vi "ADC.vi"(0 "source":tag, 1 "physical channels":tag, 2 "rate":dbl=1000.0 format="%0.2f", 3 "error in":errorcluster, 4 "samples per channel":i32=1000) -> (5 "Waveform Graph":dbl[](graph), 6 "Fourier spectrum":dbl[](graph), 7 "error out":errorcluster)   [LabVIEW 2018]
uses:
  <vilib>/DAQmx/read.llb/DAQmx Read (Analog 1D DBL 1Chan NSamp).vi
  <vilib>/DAQmx/create/channels.llb/DAQmx Create Channel (AI-Voltage-Basic).vi
  <vilib>/DAQmx/configure/timing.llb/DAQmx Timing (Sample Clock).vi
  <vilib>/DAQmx/miscellaneous.llb/DAQmx Fill In Error Info.vi
  <vilib>/Analysis/NI_AALPro.lvlib
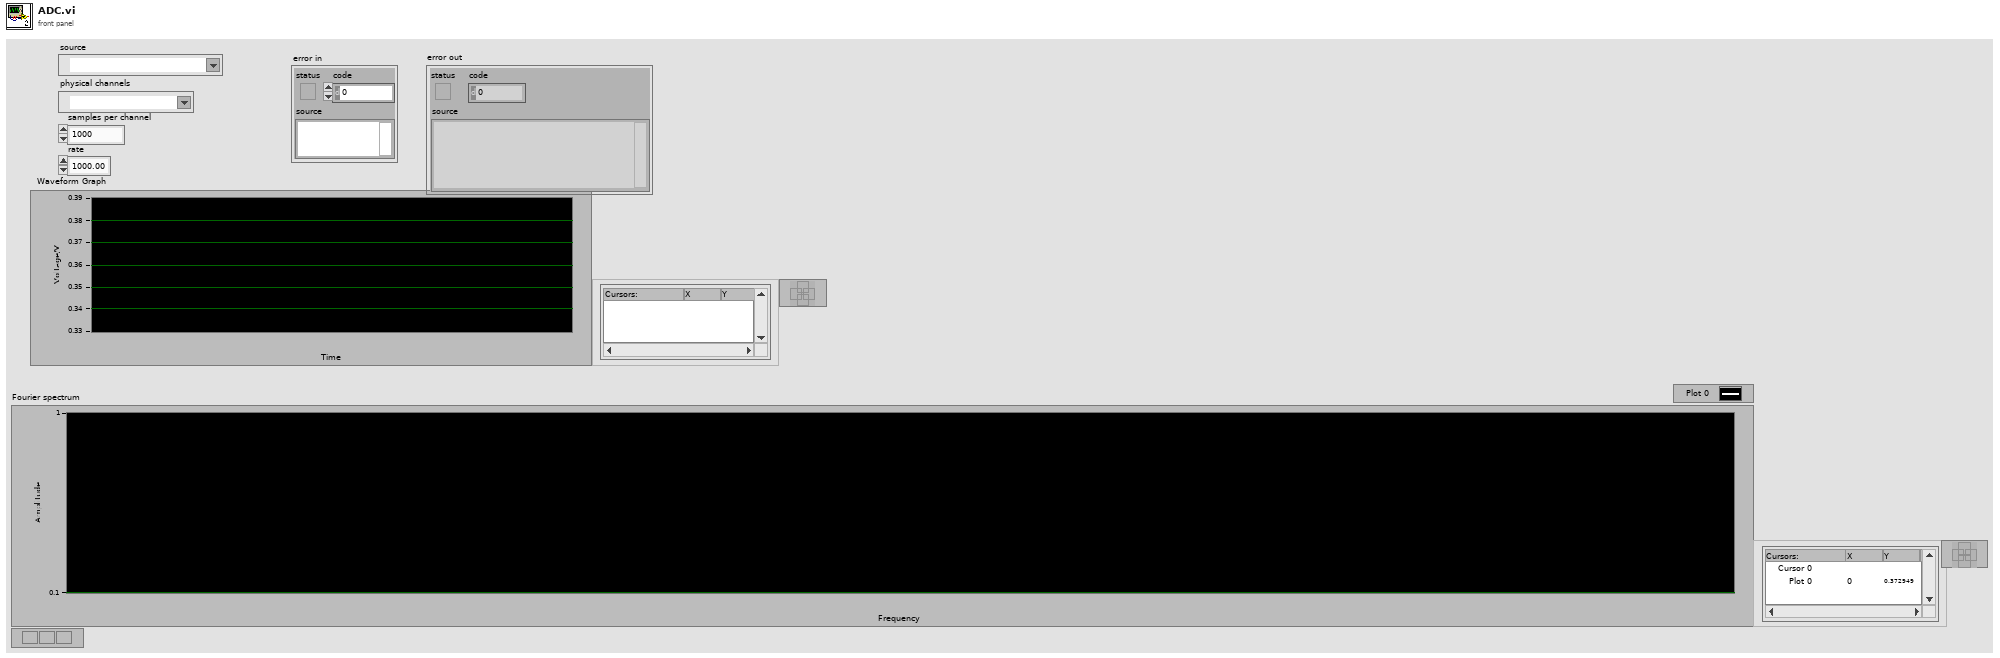
[diagram p1: front panel]
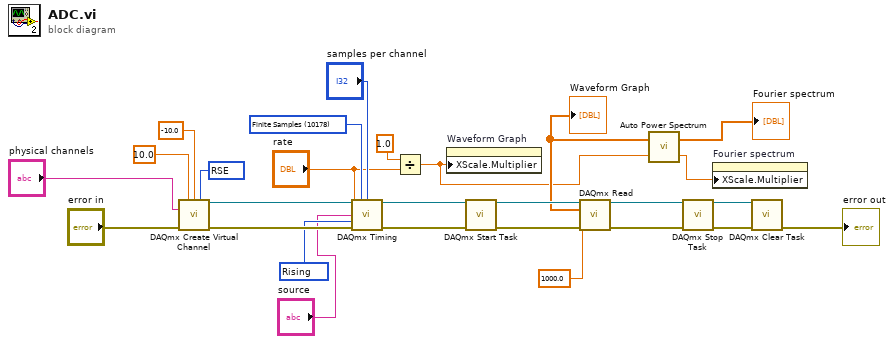
[diagram p0: block diagram]
diagram:
  w13 = 10083 items=["Default"=-1, "RSE"=10083, "NRSE"=10078, "Differential"=10106, "Pseudodifferential"=12529] ("input terminal configuration")
  w12 = 10280 items=["Rising"=10280, "Falling"=10171] ("active edge")
  w24 = 10178 items=["Finite Samples"=10178, "Continuous Samples"=10123, "Hardware Timed Single Point"=12522] ("sample mode")
  n1 = call-poly <vilib>:"DAQmx Create Virtual Channel.vi"("maximum value"=10.0, "minimum value"=-10.0, "input terminal configuration"=w13, "physical channels"="physical channels", "error in"="error in") -> ("task out"=w26:refnum<k21>, "error out"=w25:errorcluster)  [unwired: 9 in]
  n2 = call-poly <vilib>:"DAQmx Timing.vi"("task/channels in"=w26, "sample mode"=w24, "samples per channel"="samples per channel", "rate"="rate", "source"="source", "active edge"=w12, "error in"=w25) -> ("task out"=w23:refnum<k21>, "error out"=w22:errorcluster)  [unwired: 7 in]
  n3 = Divide(x=1.0, y="rate") -> (x/y=w7:dbl)
  n4 = property on="Waveform Graph" class="WFGraph (strict)"("XScale.Multiplier"=w7) -> ()  [unwired: 2 in, 2 out]
  n5 = call <vilib>:"DAQmx Start Task.vi"("task/channels in"=w23, "error in"=w22) -> ("task out"=w17:refnum<k21>, "error out"=w3:errorcluster)  [unwired: 12 in]
  n6 = call-poly <vilib>:"DAQmx Read.vi"("task/channels in"=w17, "timeout"=1000.0, "error in"=w3) -> ("task out"=w16:refnum<k21>, "data"=w8:dbl[], "error out"=w4:errorcluster)  [unwired: 10 in]
  "Waveform Graph" <- w8
  n7 = call <vilib>:"Auto Power Spectrum.vi"("dt"=w7, "Signal (V)"=w8) -> ("df"=w5:dbl, "Power Spectrum (V^2 rms)"=→"Fourier spectrum":dbl[])
  n8 = call <vilib>:"DAQmx Stop Task.vi"("task/channels in"=w16, "error in"=w4) -> ("task out"=w21:refnum<k21>, "error out"=w20:errorcluster)  [unwired: 12 in]
  n9 = property on="Fourier spectrum" class="WFGraph (strict)"("XScale.Multiplier"=w5) -> ()  [unwired: 2 in, 2 out]
  n10 = call <vilib>:"DAQmx Clear Task.vi"("task in"=w21, "error in"=w20) -> ("error out"=→"error out":errorcluster)  [unwired: 13 in]
